vi "Configure Power Analyzer.vi"(8 "error in (no error)":errorcluster, 9 "Power Analyzer Source (0: Voltage)":i32(ring) items=["Voltage", "Current"], 10 "Measurement Source (1: Main Output)":i32(ring)=1 items=["Main Output"=1, "Power Analyzer"=2], 11 "VISA resource name":refnum<visa-resource-name>) -> (0 "error out":errorcluster, 3 "VISA resource name out":refnum<visa-resource-name>)   [LabVIEW 2020, in "Agilent 681x Series.lvlib"]
doc: "Configures the measurement source to main output or power analyzer. Selects the frequency measurement source of power analyzer."
uses:
  <instrlib>/Agilent 681x Series/Agilent 681x Series.lvlib
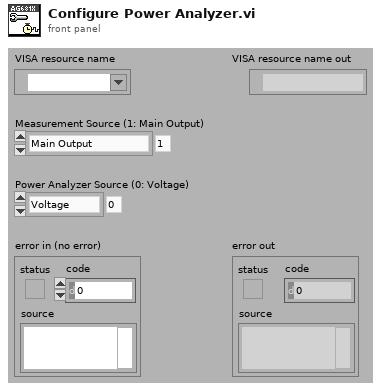
[diagram p1: front panel]
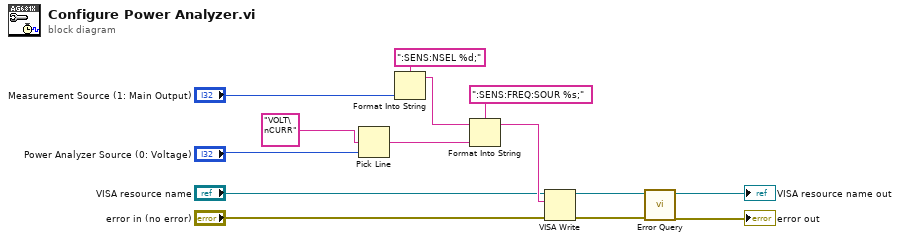
[diagram p0: block diagram]
diagram:
  n1 = Pick Line(multi-line string="VOLT\nCURR", line index="Power Analyzer Source (0: Voltage)") -> (output string=w2:string)  [unwired: 1 in]
  n2 = Format Into String(format string=":SENS:NSEL %d;", "Measurement Source (1: Main Output)") -> (resulting string=w12:string)  [unwired: 2 in, 1 out]
  n3 = Format Into String(format string=":SENS:FREQ:SOUR %s;", initial string=w12, w2) -> (resulting string=w10:string)  [unwired: 1 in, 1 out]
  n4 = VISA Write(VISA resource name="VISA resource name", write buffer=w10, error in (no error)="error in (no error)") -> (VISA resource name out=w7:refnum<visa-resource-name>, error out=w6:errorcluster)  [unwired: 1 out]
  n5 = call <instrlib>:"Error Query.vi"("error in (no error)"=w6, "VISA resource name"=w7) -> ("error out"=→"error out":errorcluster, "VISA resource name out"=→"VISA resource name out":refnum<visa-resource-name>)  [unwired: 6 in, 2 out]
